vi "ma_array_Check Time Signal Continuity (CDB).vi"(5 "Ignore input time stamp":bool, 8 "error in (no error)":errorcluster, 11 "waveforms":waveform(cdb)[](array[waveform])) -> (0 "error out":errorcluster, 1 "epsilon used":dbl[](array[numeric]) format="%0.6e", 2 "dt changed":bool[](array[boolean]), 3 "t0 changed":bool[](array[boolean]))   [LabVIEW 2020, in "NI_MABase.lvlib"]
uses:
  NI_MABase.lvlib
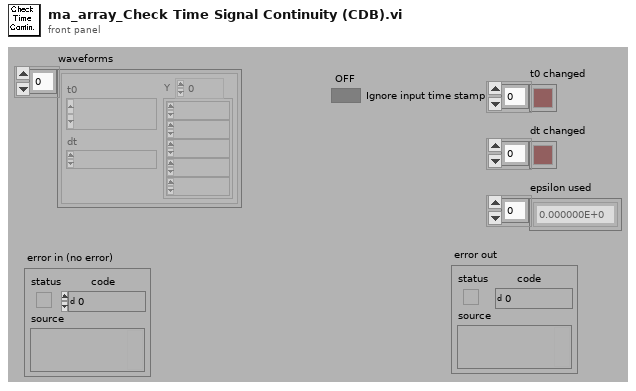
[diagram p1: front panel]
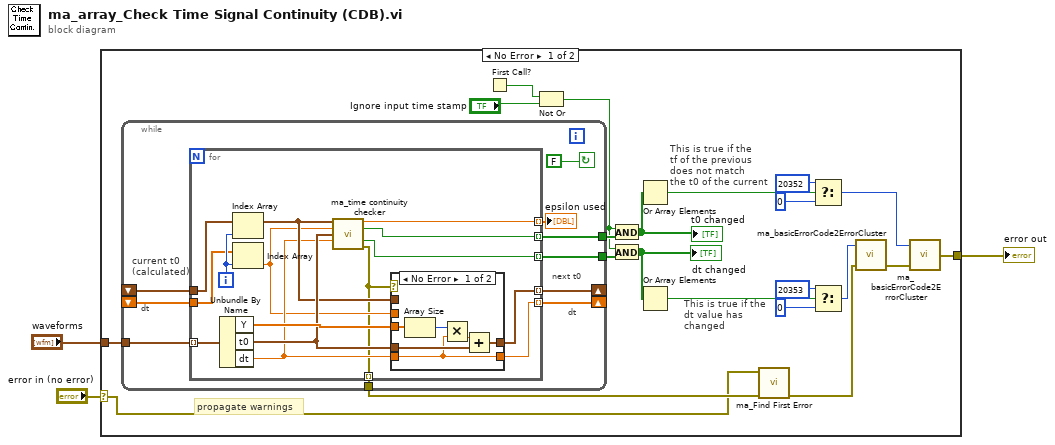
[diagram p0: block diagram]
diagram:
  n1 = case shown="No Error" "error in (no error)" {
    selector: "error in (no error)" -> [w5 w58]
    tunnel: [w11 w58] -> w2
    tunnel: "waveforms" -> [w4 _]
    frame No Error {
      # "propagate warnings"
      # "This is true if the\ntf of the previous\ndoes not match \nthe t0 of the current"
      # "This is true if the\ndt value has \nchanged"
      n2 = while {
        tunnel: [w30] -> w24
        tunnel: [w32] -> w23
        shift-left: _ -> [w31]
        shift-right: [w27] -> _
        shift-left: _ -> [w33]
        shift-right: [w34] -> _
        tunnel: [w26] -> w7
        tunnel: w4 -> [w25]
        stop <- FALSE continue-if-true
        # "current t0 \n(calculated)"
        # "dt"
        # "next t0"
        # "dt"
        n3 = for {
          tunnel: [w49] -> w34 mode=indexing
          tunnel: w33 -> [w45]
          tunnel: [w42] -> w32 mode=indexing
          tunnel: w25 -> [w47] mode=indexing
          tunnel: [w46] -> w28 mode=indexing
          tunnel: w31 -> [w38]
          tunnel: [w41] -> w30 mode=indexing
          tunnel: [w37] -> w27 mode=indexing
          tunnel: [w35] -> w26 mode=indexing
          i -> [w44]
          n4 = Unbundle By Name(w47) -> ("Y"=w48:cdb[], "t0"=w43:timestamp, "dt"=w39:dbl)
          n5 = Index Array(array=w45, index=w44) -> (element=w40:timestamp)
          n6 = Index Array(array=w38, index=w44) -> (element=w36:dbl)
          n7 = call "ma_time continuity checker.vi"("timestamp previous"=w40, "dt previous"=w36, "timestamp current"=w43, "dt current"=w39) -> ("epsilon used"=w46:dbl, "t0 changed"=w42:bool, "dt changed"=w41:bool, "error out"=w35:errorcluster)  [unwired: 8 in]
          n8 = case shown="No Error" w35 {
            tunnel: [w55 w57] -> w49
            tunnel: w48 -> [w52 _]
            tunnel: w43 -> [w51 _]
            tunnel: w40 -> [_ w57]
            tunnel: w39 -> [w50 _]
            tunnel: [w50 w56] -> w37
            tunnel: w36 -> [_ w56]
            frame No Error {
              n9 = Array Size(array=w52) -> (size(s)=w54:i32)
              n10 = Multiply(x=w54, y=w50) -> (x*y=w53:dbl)
              n11 = Add(x=w53, y=w51) -> (x+y=w55:timestamp)
            }
            frame Error {
            }
          }
        }
        "epsilon used" <- w28
      }
      n12 = First Call?() -> (First Call?: T/F=w8:bool)
      n13 = Not Or(1:"Ignore input time stamp", 2:w8) -> (0:w9:bool)
      n14 = And(x=w9, y=w23) -> (x .and. y?=w22:bool[])
      "t0 changed" <- w22
      n15 = And(x=w9, y=w24) -> (x .and. y?=w21:bool[])
      "dt changed" <- w21
      n16 = Or Array Elements(Boolean array=w22) -> (logical OR=w12:bool)
      n17 = Or Array Elements(Boolean array=w21) -> (logical OR=w13:bool)
      n18 = call "ma_Find First Error.vi"("error array in"=w7, "error in 1 (no error)"=w5) -> ("error out"=w6:errorcluster)  [unwired: 5 in]
      n19 = Select(t=20352 ("code"), s=w12, f=0) -> (s? t:f=w18:i32)
      n20 = Select(t=20353 ("code"), s=w13, f=0) -> (s? t:f=w15:i32)
      n21 = call "ma_basicErrorCode2ErrorCluster.vi"("error in (no error)"=w6, "Error Code"=w15) -> ("error out"=w14:errorcluster)  [unwired: 1 in]
      n22 = call "ma_basicErrorCode2ErrorCluster.vi"("error in (no error)"=w14, "Error Code"=w18) -> ("error out"=w11:errorcluster)  [unwired: 1 in]
    }
    frame Error {
    }
  }
  "error out" <- w2
